vi "Dbfetchrecordset.vi"() -> ()   [LabVIEW 2019]
uses:
  <vilib>/addons/database/NI_Database_API.lvlib
  <vilib>/addons/database/Auxilliary.llb/DB Tools Cursor Type.ctl
  <vilib>/addons/database/Recordset.llb/Rec Get Recordset Properties (R).vi
  <vilib>/addons/database/Recordset.llb/Rec Destroy - Connection.vi
  <vilib>/addons/database/Recordset.llb/Rec Fetch Next Recordset (R).vi
  <vilib>/addons/database/Recordset.llb/Rec Move To Next Record (R).vi
  <vilib>/addons/database/Connection.llb/Conn Execute.vi
  <vilib>/addons/database/Connection.llb/DB Tools Open Connec (String).vi
panel:
  in  "Next Record":bool
  in  "Stop  Opreation":bool
  in  "Provide your ODBC server":string
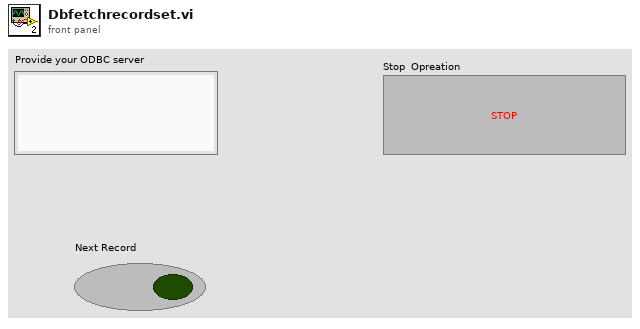
[diagram p1: front panel]
types:
  T1 = typedef "NI_Database_API.lvlib/DB Tools Cursor Type.ctl" = enum16{"forward-only", "keyset", "dynamic", "static"}
  T2 = typedef "NI_Database_API.lvlib/Conn ObjectReference.ctl" = refnum<k1>
  T3 = typedef "NI_Database_API.lvlib/Rec ObjectReference.ctl" = refnum<k1>
  T4 = typedef "NI_Database_API.lvlib/Rec Properties.ctl" = cluster{"column count":i32, "record index":i32, "record count":i32, "bof?":bool, "eof?":bool, "cursor type":T1, "cache size":i32, "state":enum16{"closed", "open"}}
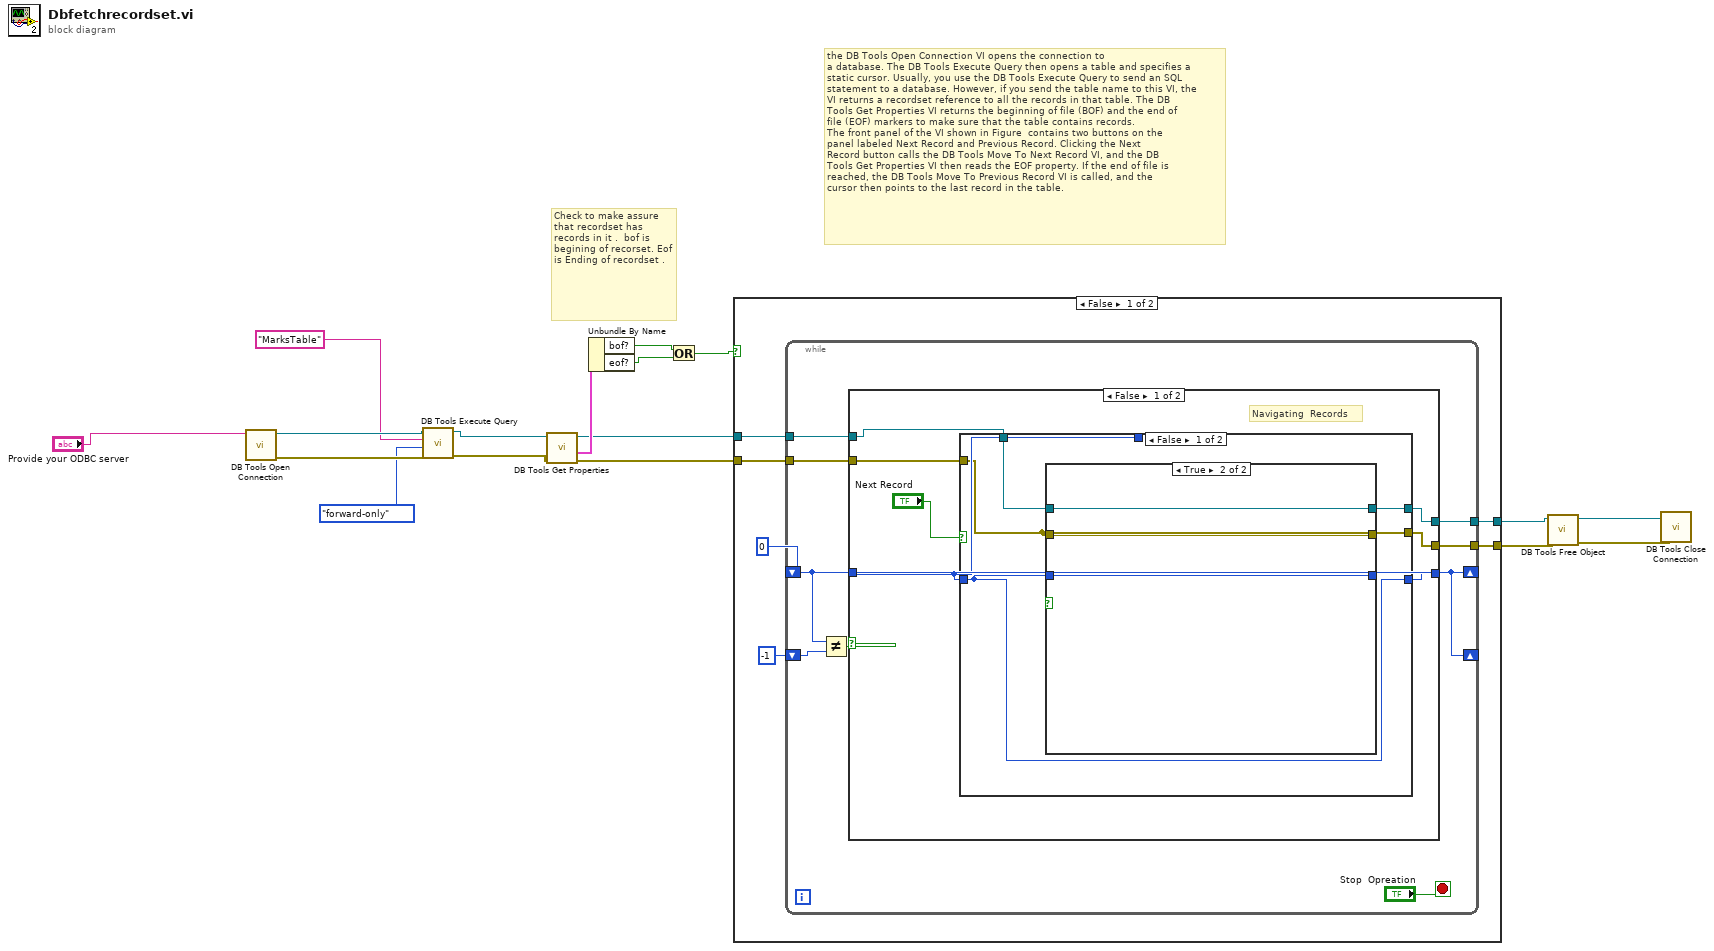
[diagram p0: block diagram]
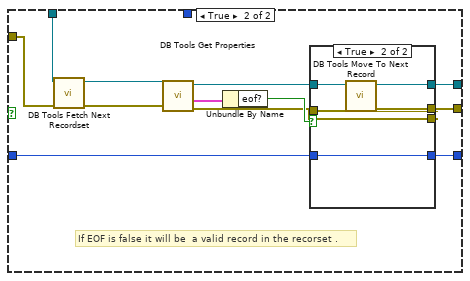
[diagram p3: hidden frame]
diagram:
  # "the DB Tools Open Connection VI opens the connection to\na database. The DB Tools Execute Query then opens a table and specifies a\nstatic cursor. Usually, you use the DB Tools Execute Query to send an SQL\nstatement to a database. However, if you send the table name to this VI, the\nVI returns a recordset reference to all the records in that table. The DB\nTools Get Properties VI returns the beginning of file (BOF) and the end of\nfile (EOF) markers to make sure that the table contains records.\nThe front panel of the VI shown in Figure  contains two buttons on the\npanel labeled Next Record and Previous Record. Clicking the Next\nRecord button calls the DB Tools Move To Next Record VI, and the DB\nTools Get Properties VI then reads the EOF property. If the end of file is\nreached, the DB Tools Move To Previous Record VI is called, and the\ncursor then points to the last record in the table."
  # "Check to make assure that recordset has records in it .  bof is begining of recorset. Eof is Ending of recordset ."
  n1 = call-poly <vilib>:"DB Tools Open Connection.vi"("connection information"="Provide your ODBC server") -> ("error out"=w15:errorcluster, "connection reference"=w16:T2)  [unwired: 7 in]
  n2 = call-poly <vilib>:"DB Tools Execute Query.vi"("error in (no error)"=w15, "cursor type"=DB_Tools_Cursor_Type."forward-only", "SQL query"="MarksTable", "connection reference"=w16) -> ("error out"=w11:errorcluster, "recordset reference"=w12:T3)  [unwired: 4 in]
  n3 = call-poly <vilib>:"DB Tools Get Properties.vi"("error in (no error)"=w11, "recordset reference"=w12) -> ("error out"=w1:errorcluster, "recordset properties"=w10:T4, "recordset reference out"=w6:T3)  [unwired: 3 in]
  n4 = Unbundle By Name(w10) -> ("bof?"=w9:bool, "eof?"=w8:bool)
  n5 = Or(x=w9, y=w8) -> (x .or. y?=w7:bool)
  n6 = case shown="False" w7 {
    tunnel: w6 -> [w21 w69]
    tunnel: [w20 w69] -> w5
    tunnel: [w19 w68] -> w4
    tunnel: w1 -> [w18 w68]
    frame False {
      n7 = while {
        shift-right: [w24] -> _
        shift-left: 0 -> [w24]
        shift-right: [w24] -> _
        shift-left: -1 -> [w30]
        tunnel: w21 -> [w28]
        tunnel: [w27] -> w20
        tunnel: [w26] -> w19
        tunnel: w18 -> [w25]
        stop <- "Stop  Opreation" stop-if-true
        n8 = Not Equal?(x=w24, y=w30) -> (x != y?=w29:bool)
        n9 = case shown="False" w29 {
          tunnel: w28 -> [w37 w66]
          tunnel: [w36 w66] -> w27
          tunnel: [w35 w65] -> w26
          tunnel: w24 -> [w34 w67]
          tunnel: [w33 w67] -> _
          tunnel: w25 -> [w32 w65]
          frame False {
            # "Navigating  Records"
            n10 = case shown="False" "Next Record" {
              tunnel: w37 -> [w41 w56]
              tunnel: [w41 w49] -> w36
              tunnel: [w40 w48] -> w35
              tunnel: w34 -> [_ _]
              tunnel: w34 -> [w39 w47]
              tunnel: [w39 w46] -> w33
              tunnel: w32 -> [w40 w45]
              frame False {
                n11 = case shown="True" {
                  selector: _ -> [_ _]
                  tunnel: [_ w44] -> _
                  tunnel: w41 -> [_ w44]
                  tunnel: [_ w43] -> _
                  tunnel: w40 -> [_ w43]
                  tunnel: w39 -> [_ w42]
                  tunnel: [_ w42] -> _
                  frame False {
                  }
                  frame True {
                  }
                }
              }
              frame True {
                # "If EOF is false it will be  a valid record in the recorset ."
                n12 = call-poly <vilib>:"DB Tools Fetch Next Recordset.vi"("error in (no error)"=w45, "recordset reference"=w56) -> ("error out"=w55:errorcluster, "recordset reference out"=w54:T3)  [unwired: 4 in]
                n13 = call-poly <vilib>:"DB Tools Get Properties.vi"("error in (no error)"=w55, "recordset reference"=w54) -> ("error out"=w50:errorcluster, "recordset properties"=w53:T4, "recordset reference out"=w51:T3)  [unwired: 3 in]
                n14 = Unbundle By Name(w53) -> ("eof?"=w52:bool)
                n15 = case shown="True" w52 {
                  tunnel: w51 -> [w59 w64]
                  tunnel: w50 -> [w57 w60]
                  tunnel: [w59 w63] -> w49
                  tunnel: [w57 w62] -> w48
                  tunnel: [w58 w61] -> w46
                  tunnel: w47 -> [w58 w61]
                  tunnel: [w57 w60] -> _
                  frame False {
                  }
                  frame True {
                    n16 = call-poly <vilib>:"DB Tools Move To Next Record.vi"("error in (no error)"=w60, "recordset reference"=w64) -> ("error out"=w62:errorcluster, "recordset reference out"=w63:T3)  [unwired: 8 in]
                  }
                }
              }
            }
          }
          frame True {
          }
        }
      }
    }
    frame True {
    }
  }
  n17 = call-poly <vilib>:"DB Tools Free Object.vi"("error in (no error)"=w4, "recordset reference"=w5) -> ("error out"=w2:errorcluster, "connection reference"=w3:T2)  [unwired: 8 in]
  n18 = call <vilib>:"DB Tools Close Connection.vi"("error in (no error)"=w2, "connection reference"=w3) -> ()  [unwired: 5 in, 1 out]
